vi "Shut Down Device.vi"(8 "error in (no error)":errorcluster, 11 "Alltesta Autosampler in":refnum<class "Alltesta Autosampler.lvclass">) -> (0 "error out":errorcluster, 3 "Alltesta Autosampler out":refnum<class "Alltesta Autosampler.lvclass">)   [LabVIEW 2023, in "Alltesta Autosampler.lvlib" / "Alltesta Autosampler.lvclass"]
uses:
  Alltesta Autosampler.lvclass
  Alltesta Autosampler.lvclass/Alltesta Autosampler.ctl
  Autosampler/Autosampler.lvclass
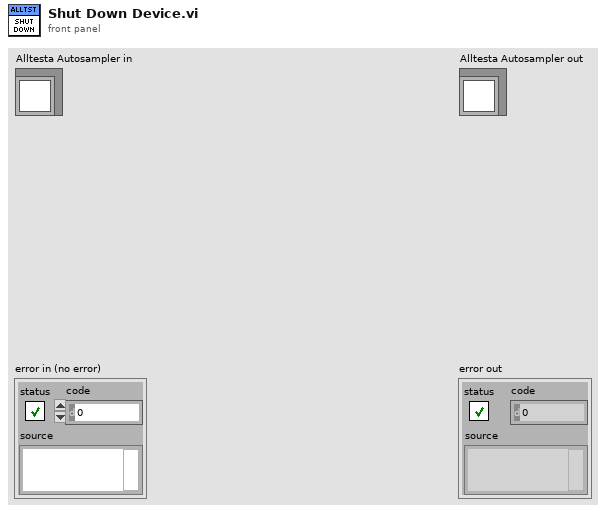
[diagram p1: front panel]
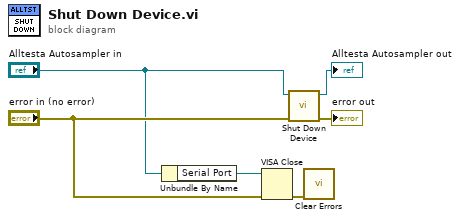
[diagram p0: block diagram]
diagram:
  n1 = Unbundle By Name("Alltesta Autosampler in") -> ("Serial Port"=w1:refnum<visa-resource-name>)
  n2 = VISA Close(VISA resource name=w1, error in (no error)="error in (no error)") -> (error out=w4:errorcluster)
  n3 = call-parent "Shut Down Device.vi"("error in (no error)"="error in (no error)", "Device in"="Alltesta Autosampler in") -> ("error out"=→"error out":errorcluster, "Device out"=→"Alltesta Autosampler out":refnum<class "Alltesta Autosampler.lvclass">)  [unwired: 8 in]
  n4 = call <vilib>:"Clear Errors.vi"("error in (no error)"=w4) -> ()  [unwired: 5 in, 2 out]
